vi "WS_InsertProcessDataWithFails.vi"(0 "PassFail":i32, 2 "EndTime":string, 3 "EntryTime":string, 4 "FailString":string, 5 "ProcessName":string, 6 "StationName":string, 7 "SerialNumber":string) -> (1 "Reply":string)   [LabVIEW 2022 SP3]
uses:
  C:/Users/K90011729/OneDrive - Kimball Electronics/Desktop/Proyectos/IPB2 Test secuence/WsConnector/WSConnector.dll
  WSConnector.dll
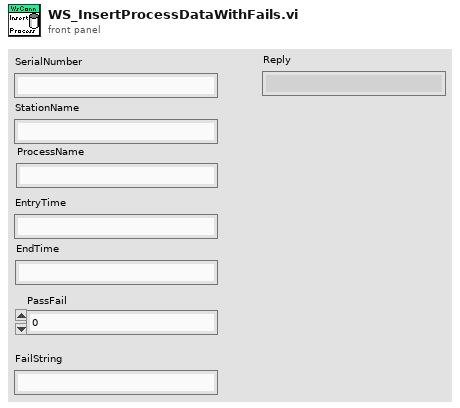
[diagram p1: front panel]
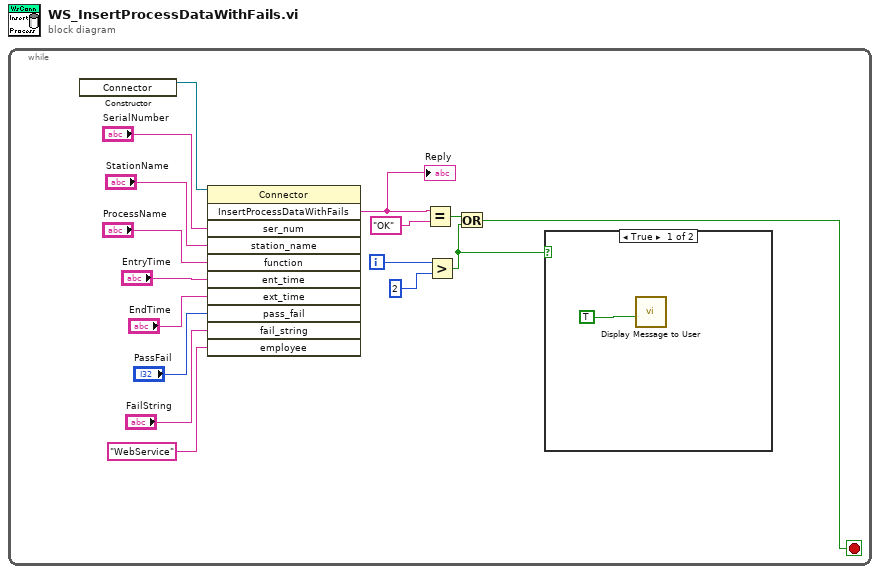
[diagram p0: block diagram]
diagram:
  n1 = while {
    i -> [w2]
    stop <- w4 stop-if-true
    n2 = constructor class="Connector"() -> (reference out=w1:refnum<k24>)  [unwired: 3 in, 2 out]
    n3 = invoke class="Connector" method="InsertProcessDataWithFails"(reference=w1, "ser_num"="SerialNumber", "station_name"="StationName", "function"="ProcessName", "ent_time"="EntryTime", "ext_time"="EndTime", "pass_fail"="PassFail", "fail_string"="FailString", "employee"="WebService") -> ("InsertProcessDataWithFails"=w3:string)  [unwired: 2 in, 10 out]
    "Reply" <- w3
    n4 = Equal?(x=w3, y="OK") -> (x = y?=w5:bool)
    n5 = Greater?(x=w2, y=2) -> (0:w6:bool)
    n6 = Or(x=w5, y=w6) -> (x .or. y?=w4:bool)
    n7 = case shown="True" w6 {
      frame True {
        n8 = call "Display Message to User"("Enable"=TRUE) -> ()  [unwired: 9 in, 2 out]
      }
      frame False {
      }
    }
  }
